vi "DriveModuleControl_TravTuneKsKv.vi"(8 "error in":errorcluster, 9 "Actual State":T1={"Speed"=0.0, "Angle"={"VALUE"=0.0, "COS"=1.0, "SIN"=0.0}} {"Angle"."SIN" format="%13.4f"; "Angle"."COS" format="%13.4f"; "Angle"."VALUE" format="%13.4f"}, 10 "Desired State":T1={"Speed"=0.0, "Angle"={"VALUE"=0.0, "COS"=1.0, "SIN"=0.0}} {"Angle"."SIN" format="%13.4f"; "Angle"."COS" format="%13.4f"; "Angle"."VALUE" format="%13.4f"}, 11 "ModualNamePrefix":i32) -> (0 "error out":errorcluster)   [LabVIEW 2020]
uses:
  <vilib>/Rock Robotics/WPI/ThirdParty/JAS_Junk/TrajLib/TypeDef/SWERVE_DRIVE_MODULE_STATE.ctl
  <vilib>/Rock Robotics/WPI/ThirdParty/JAS_Junk/TrajLib/TypeDef/ROTATION2D.ctl
  <vilib>/Rock Robotics/WPI/ThirdParty/JAS_Junk/TrajLib/Rotation2d_Minus.vi
  <vilib>/Rock Robotics/WPI/ThirdParty/JAS_Junk/TrajLib/Rotation2d_GetRadians.vi
  <vilib>/Rock Robotics/WPI/ThirdParty/JAS_Junk/TrajLib/SwerveModuleState_New.vi
  <vilib>/Rock Robotics/WPI/ThirdParty/JAS_Junk/TrajLib/Rotation2d_RotateBy.vi
  <vilib>/Rock Robotics/WPI/ThirdParty/JAS_Junk/TrajLib/Rotation2d_CreateAngle.vi
  <vilib>/Rock Robotics/WPI/ThirdParty/JAS_Junk/TrajLib/SimpleMotorFF_Calculate.vi
  <vilib>/Rock Robotics/WPI/ThirdParty/JAS_Junk/TrajLib/PIDController_AtSetpoint.vi
  <vilib>/Rock Robotics/WPI/ThirdParty/JAS_Junk/TrajLib/PIDController_SetPIDF.vi
  <vilib>/Rock Robotics/WPI/ThirdParty/JAS_Junk/TrajLib/PIDController_SetDerivativeFilter.vi
  <vilib>/Rock Robotics/WPI/ThirdParty/JAS_Junk/TrajLib/PIDController_SetIntegratorRange.vi
  <vilib>/Rock Robotics/WPI/ThirdParty/JAS_Junk/TrajLib/PIDController_SetTolerancePandV.vi
  <vilib>/Rock Robotics/WPI/ThirdParty/JAS_Junk/TrajLib/PIDController_DisableContinousInput.vi
  <vilib>/Rock Robotics/WPI/ThirdParty/JAS_Junk/TrajLib/PIDController_EnableContinousInput.vi
  <vilib>/Rock Robotics/WPI/ThirdParty/JAS_Junk/TrajLib/PIDController_Reset.vi
  <vilib>/Rock Robotics/WPI/ThirdParty/JAS_Junk/TrajLib/PIDController_New.vi
  <vilib>/Rock Robotics/WPI/ThirdParty/JAS_Junk/TrajLib/PIDController_SetOutputLimits.vi
  <vilib>/Rock Robotics/WPI/ThirdParty/JAS_Junk/TrajLib/LinearFilter_ResetToValue.vi
  <vilib>/Rock Robotics/WPI/ThirdParty/JAS_Junk/TrajLib/LinearFilter_Calculate.vi
  <vilib>/Rock Robotics/WPI/ThirdParty/JAS_Junk/TrajLib/Rotation2d_UnaryMinus.vi
  <vilib>/Rock Robotics/WPI/ThirdParty/JAS_Junk/TrajLib/Rotation2d_CreateXY.vi
  <vilib>/Rock Robotics/WPI/ThirdParty/JAS_Junk/TrajLib/PIDController_NewPeriod.vi
  <vilib>/Rock Robotics/WPI/ThirdParty/JAS_Junk/TrajLib/Util_CalcDist.vi
  <vilib>/Rock Robotics/SystemInterfaces/NetworkCommunication/NetComm_UsageReport_report.vi
  DriveGlobal.vi
  <vilib>/Rock Robotics/WPI/ThirdParty/JAS_Junk/TrajLib/LinearFilter_MovingAverage.vi
  <vilib>/Rock Robotics/WPI/ThirdParty/JAS_Junk/TrajLib/LinearFilter_LowPassBW1.vi
  <vilib>/Rock Robotics/WPI/ThirdParty/JAS_Junk/TrajLib/LinearFilter_LowPassBW2.vi
  <vilib>/Rock Robotics/WPI/ThirdParty/JAS_Junk/TrajLib/LinearFilter_HighPassBW1.vi
  <vilib>/Rock Robotics/WPI/ThirdParty/JAS_Junk/TrajLib/LinearFilter_HighPassBW2.vi
  <vilib>/Rock Robotics/WPI/ThirdParty/JAS_Junk/TrajLib/Globals/Util_LibraryGlobals.vi
  <vilib>/Rock Robotics/WPI/ThirdParty/JAS_Junk/TrajLib/PIDController_AdvCalculate_FF_Sp_Pv.vi
  <vilib>/Utility/semaphor.llb/Obtain Semaphore Reference.vi
  <vilib>/Rock Robotics/WPI/ThirdParty/JAS_Junk/TrajLib/Timer_Reset.vi
  <vilib>/Rock Robotics/Network Tables/NT Write Number.vi
  <vilib>/Rock Robotics/WPI/ThirdParty/JAS_Junk/TrajLib/Trajectory_Library.lvlib
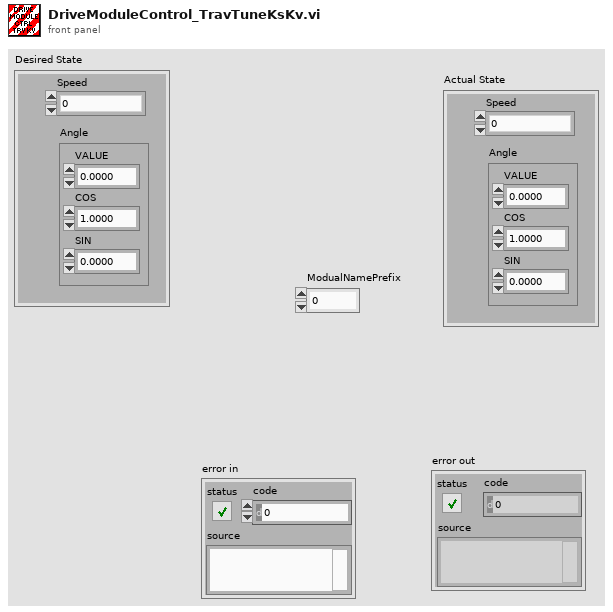
[diagram p1: front panel]
types:
  T1 = typedef "Trajectory_Library.lvlib/SWERVE_DRIVE_MODULE_STATE.ctl" = cluster{"Speed":dbl, "Angle":T2}
  T2 = typedef "Trajectory_Library.lvlib/ROTATION2D.ctl" = cluster{"VALUE":dbl, "COS":dbl, "SIN":dbl}
  T3 = enum16{"Moving Average", "Low Pass 1st Order Butterworth", "Low Pass 2nd Order Butterworth", "High Pass 1st Order Butterworth", "High Pass 2nd Order Butterworth"}
  T4 = typedef "WPI_MotorControlDeviceRef.ctl" = cluster{"DeviceStatus":errorcluster, "Type":T5, "PWM":cluster{"PWM Channel":T6, "DeadBand":T7}, "CAN":cluster{"Device Number":u8, "SetOutput VI Ref":variant, "GetOutput VI Ref":variant, "Enable VI Ref":variant, "Disable VI Ref":variant, "Data":variant}, "Invert":bool, "DIO PWM":cluster{"PWM \"Enable\" Channel":T6, "DIOChannel":T8, "PWM Rate":dbl}}
  T5 = typedef "WPI_MotorControlType.ctl" = enum16{"PWM", "CAN", "DIO PWM"}
  T6 = typedef "FPGA_DIOPWMChannel.ctl" = enum8{"PWM 0", "PWM 1", "PWM 2", "PWM 3", "PWM 4", "PWM 5", "PWM 6", "PWM 7", "PWM 8", "PWM 9", "PWM MXP 0", "PWM MXP 1", "PWM MXP 2", "PWM MXP 3", "PWM MXP 4", "PWM MXP 5", "PWM MXP 6", "PWM MXP 7", "PWM MXP 8", "PWM MXP 9", "Invalid"}
  T7 = typedef "WPI_PWMDeadband.ctl" = cluster{"Name":string, "maxPositivePwm":i32, "minPositivePwm":i32, "centerPwm":i32, "maxNegativePwm":i32, "minNegativePwm":i32, "angularRange":u16}
  T8 = typedef "FPGA_DIOChannel.ctl" = enum8{"DIO 0", "DIO 1", "DIO 2", "DIO 3", "DIO 4", "DIO 5", "DIO 6", "DIO 7", "DIO 8", "DIO 9", "DIO MXP 0", "DIO MXP 1", "DIO MXP 2", "DIO MXP 3", "DIO MXP 4", "DIO MXP 5", "DIO MXP 6", "DIO MXP 7", "DIO MXP 8", "DIO MXP 9", "DIO MXP 10", "DIO MXP 11", "DIO MXP 12", "DIO MXP 13", "DIO MXP 14", "DIO MXP 15", "SPI Port CS1", "SPI Port CS2", "SPI Port CS3", "SPI Port MISO", "SPI Port MOSI", "Invalid"}
  T9 = typedef "Trajectory_Library.lvlib/TIMER.ctl" = cluster{"StartTime":dbl, "Accumulated TIme":dbl, "Running":bool, "semaphore":T10}
  T10 = typedef "Semaphore RefNum" = refnum<k1>
  T11 = typedef "Trajectory_Library.lvlib/SIMPLE_MOTOR_FF.ctl" = cluster{"Ks":dbl, "Kv":dbl, "Ka":dbl, "KnInv":dbl}
  T12 = typedef "Trajectory_Library.lvlib/PID_ADV_LIMITS.ctl" = cluster{"MaxInput":dbl, "MinInput":dbl, "Continuous":bool, "MaxOutput":dbl, "MinOutput":dbl}
  T13 = typedef "Trajectory_Library.lvlib/PID_ADV_TUNING.ctl" = cluster{"Kf":dbl, "Kp":dbl, "Ki":dbl, "Kd":dbl, "MaximumIntegral":dbl, "MinimumIntegral":dbl, "Filter Derivative":bool}
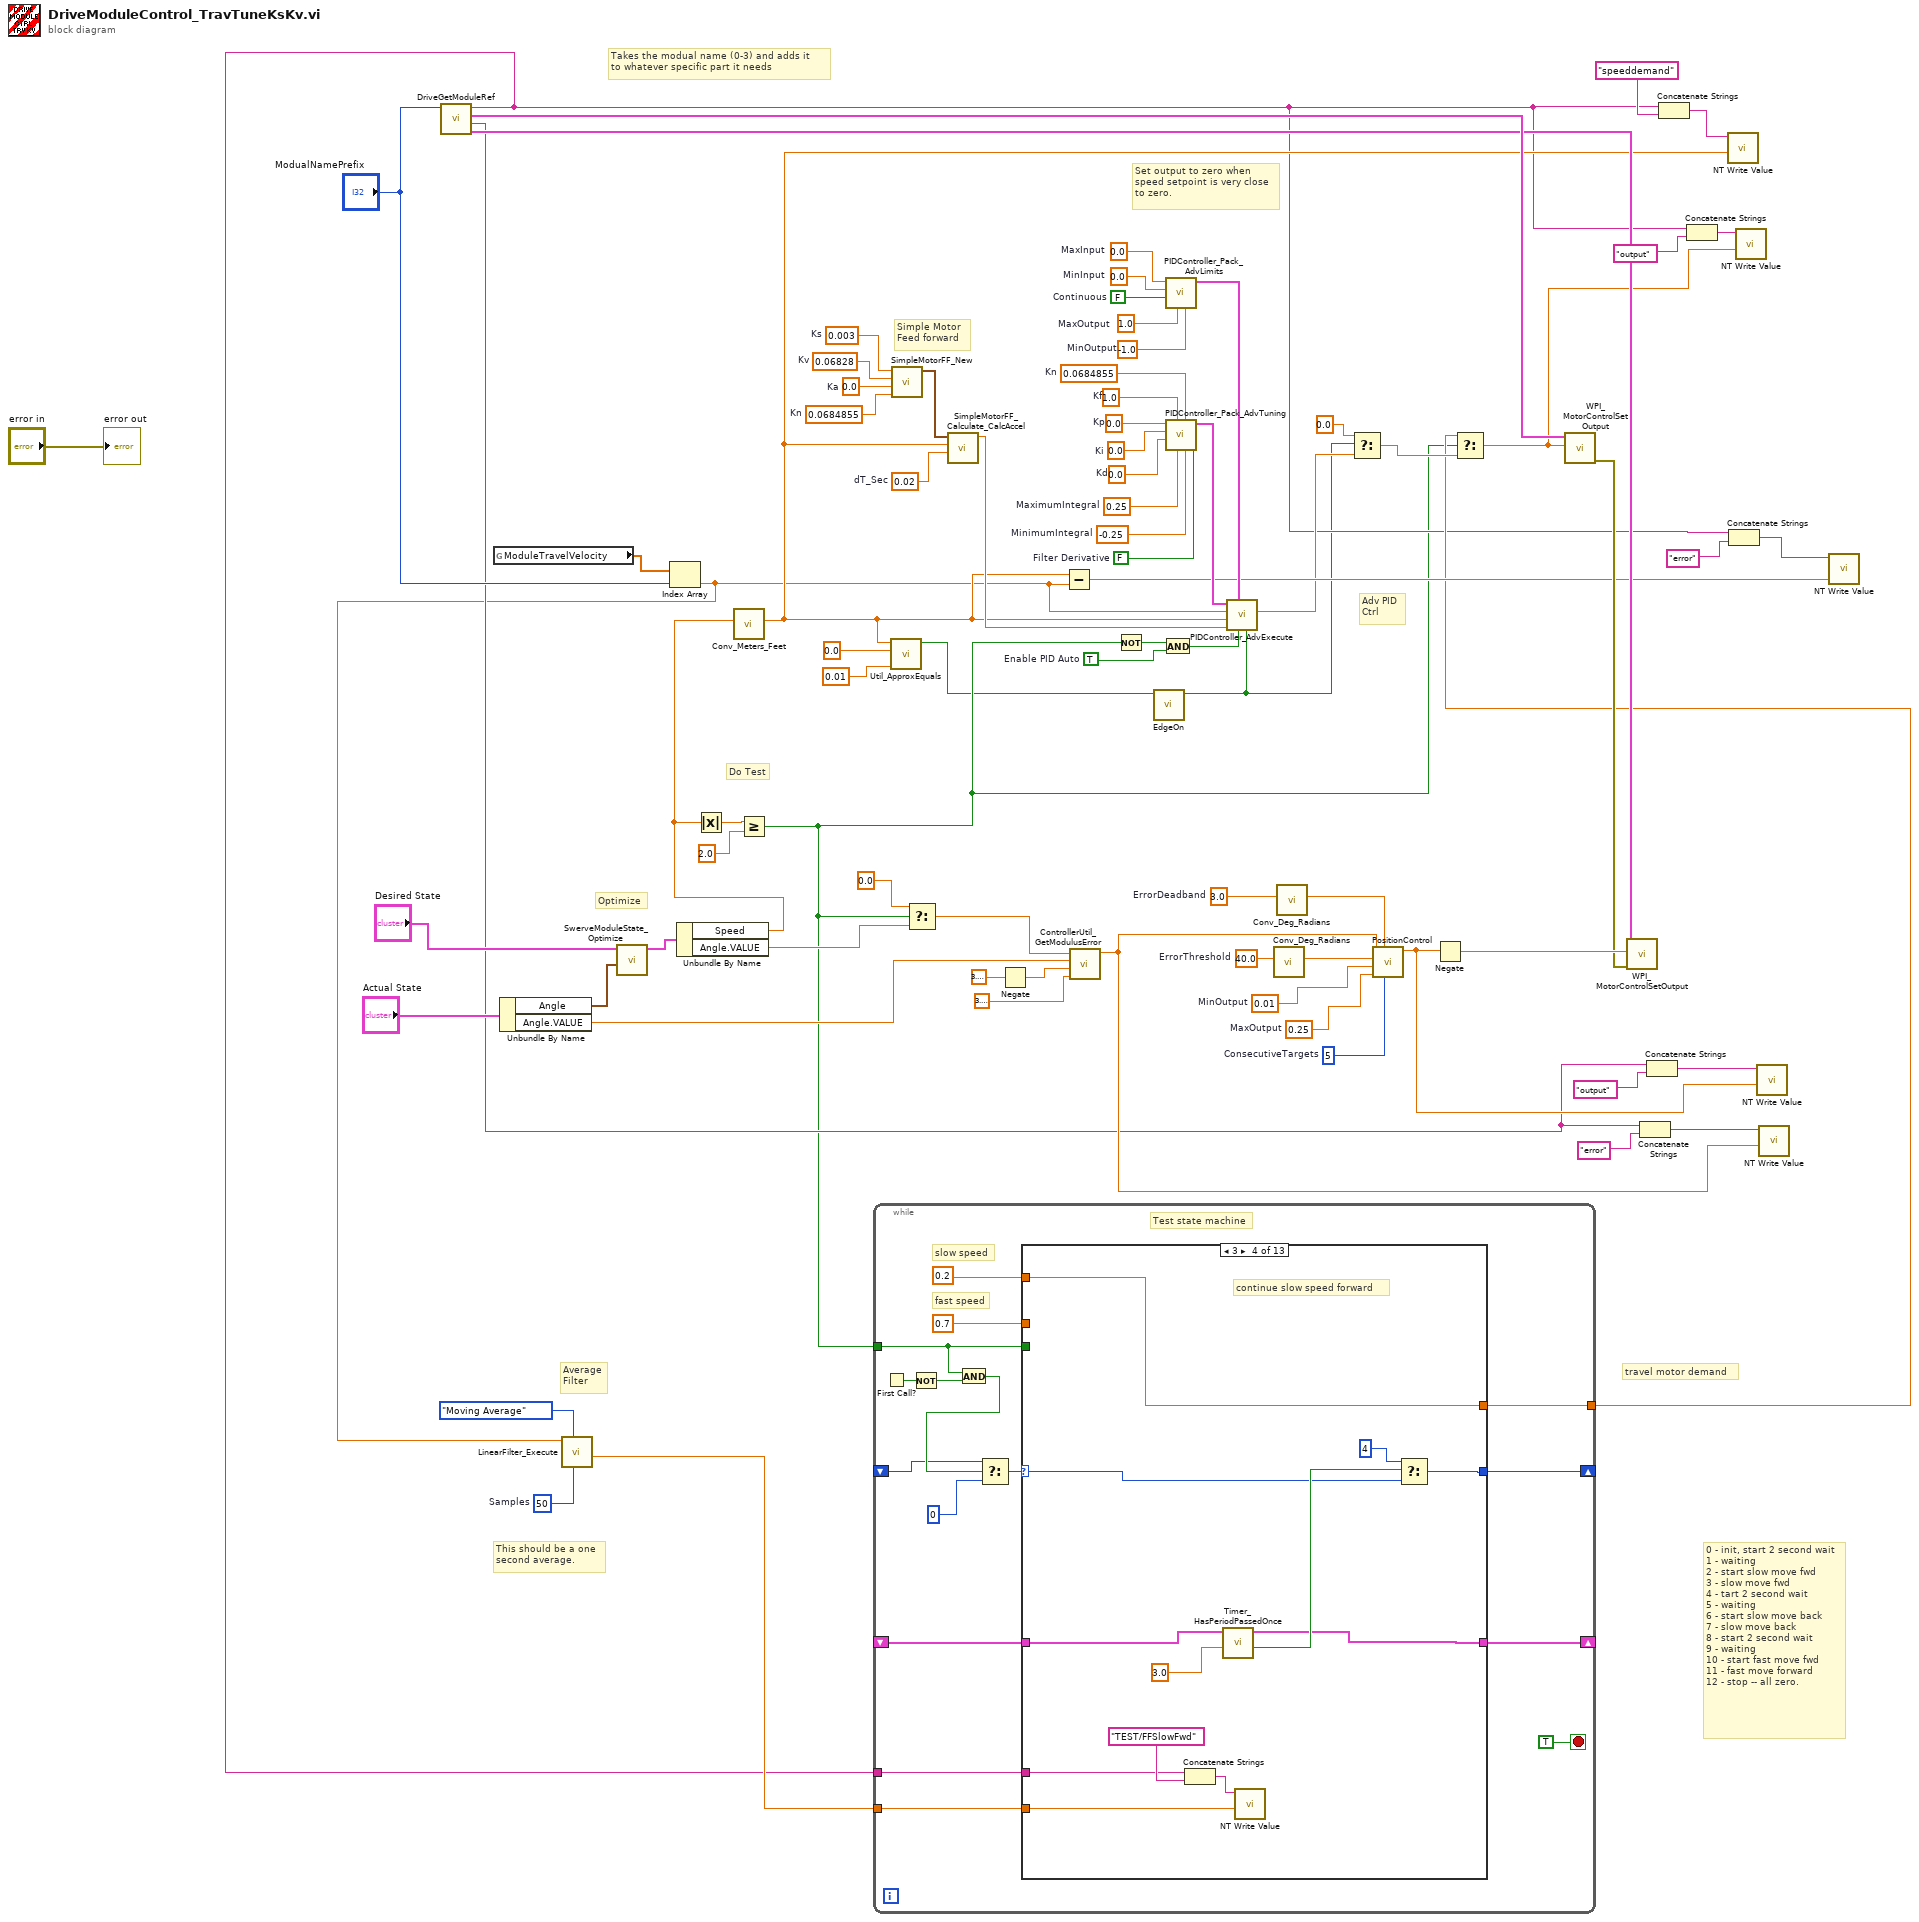
[diagram p0: block diagram]
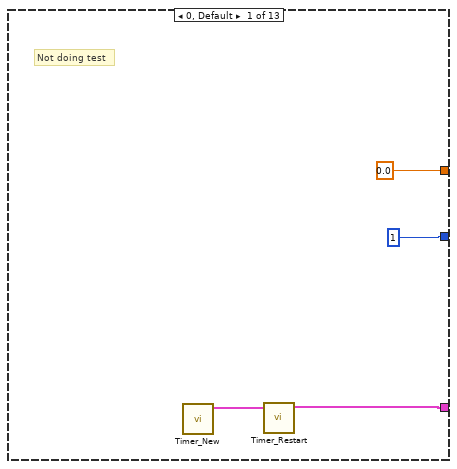
[diagram p2: hidden frame]
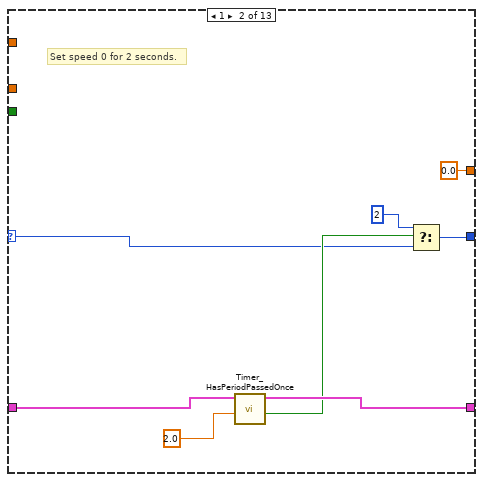
[diagram p3: hidden frame]
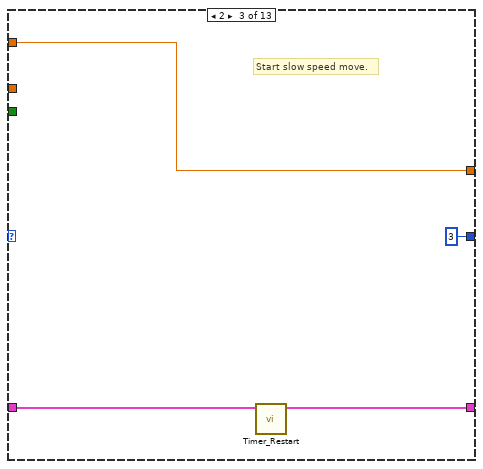
[diagram p4: hidden frame]
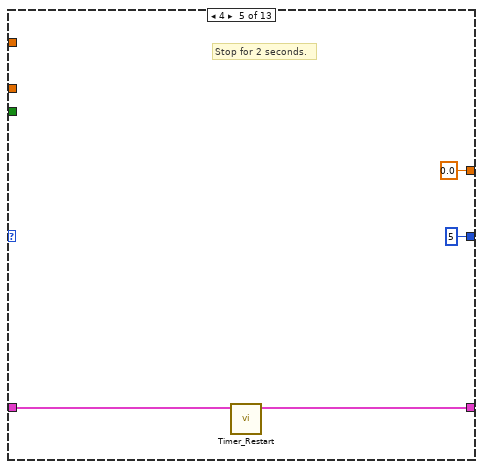
[diagram p5: hidden frame]
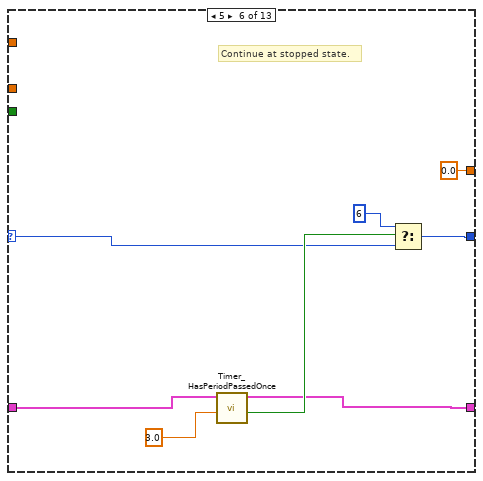
[diagram p6: hidden frame]
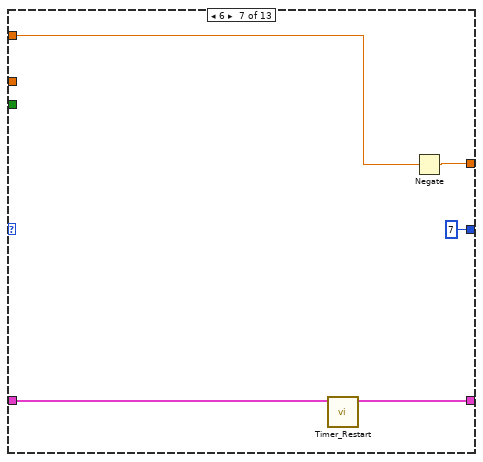
[diagram p7: hidden frame]
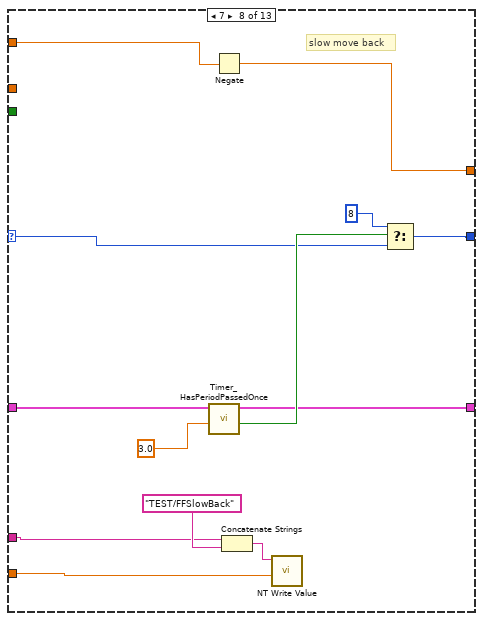
[diagram p8: hidden frame]
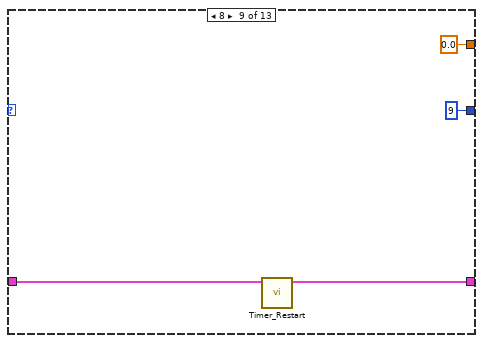
[diagram p9: hidden frame]
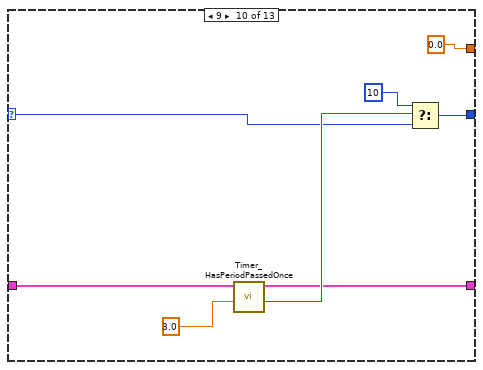
[diagram p10: hidden frame]
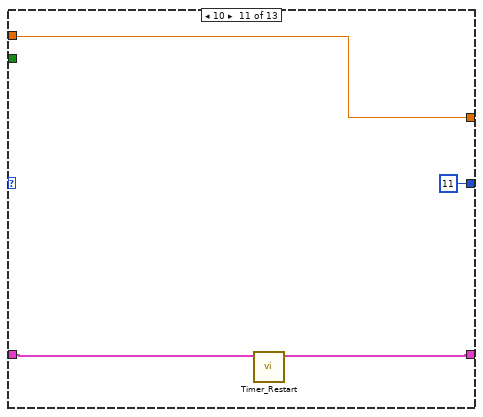
[diagram p11: hidden frame]
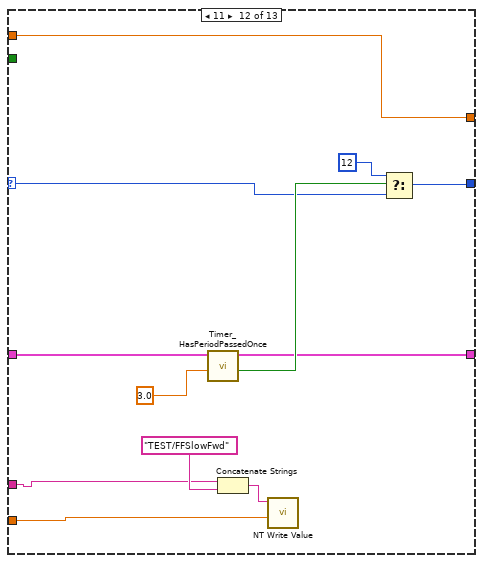
[diagram p12: hidden frame]
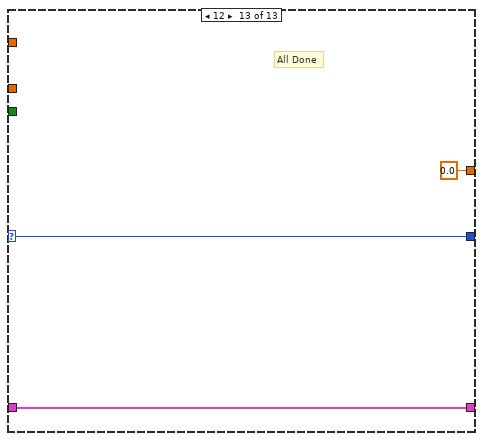
[diagram p13: hidden frame]
diagram:
  w8 = 50  # Samples
  w20 = TRUE  # Enable PID Auto
  w30 = 0.0684855  # Kn
  w47 = 0.0  # Kp
  w46 = 0.0  # Ki
  w45 = 0.0  # Kd
  w44 = 1.0  # Kf
  w43 = 0.25  # MaximumIntegral
  w42 = -0.25  # MinimumIntegral
  w41 = FALSE  # Filter Derivative
  w39 = 0.0  # MinInput
  w38 = FALSE  # Continuous
  w37 = 1.0  # MaxOutput
  w40 = -1.0  # MinOutput
  w36 = 0.0  # MaxInput
  w56 = 0.0684855  # Kn
  w55 = 0.02  # dT_Sec
  w53 = 0.003  # Ks
  w52 = 0.06828  # Kv
  w51 = 0.0  # Ka
  w66 = 5  # ConsecutiveTargets
  w63 = 0.25  # MaxOutput
  w67 = 0.01  # MinOutput
  w60 = 40.0  # ErrorThreshold
  w62 = 3.0  # ErrorDeadband
  # "This should be a one\nsecond average."
  # "Average\nFilter"
  # "0 - init, start 2 second wait\n1 - waiting\n2 - start slow move fwd\n3 - slow move fwd\n4 - tart 2 second wait\n5 - waiting\n6 - start slow move back\n7 - slow move back\n8 - start 2 second wait\n9 - waiting\n10 - start fast move fwd\n11 - fast move forward\n12 - stop -- all zero."
  # "travel motor demand"
  # "Do Test"
  # "Optimize"
  # "Set output to zero when\nspeed setpoint is very close\nto zero."
  # "Adv PID\nCtrl"
  # "Simple Motor\nFeed forward"
  # "Takes the modual name (0-3) and adds it \nto whatever specific part it needs"
  n1 = call "DriveGetModuleRef.vi"("ModualNamePrefix"="ModualNamePrefix") -> ("SpinMot"=w48:T4, "SpinStr"=w26:string, "TravMot"=w49:T4, "TravStr"=w4:string)  [unwired: 5 in, 2 out]
  n2 = global read "DriveGlobal.vi" "ModuleTravelVelocity"() -> (w32:dbl[])
  n3 = Unbundle By Name("Actual State") -> ("Angle"=w73:T2, "Angle.VALUE"=w70:dbl)
  n4 = call <vilib>:"SwerveModuleState_Optimize.vi"("CurrentAngle"=w73, "Desired State"="Desired State") -> ("out SWERVE_DRIVE_MODULE_STATE"=w71:T1)  [unwired: 9 in]
  n5 = Index Array(array=w32, index="ModualNamePrefix") -> (element=w6:dbl)
  n6 = call <vilib>:"LinearFilter_Execute.vi"("Samples"=w8, "Filter Type"=T3."Moving Average", "Input"=w6) -> ("Output"=w5:dbl)  [unwired: 7 in, 1 out]
  n7 = Unbundle By Name(w71) -> ("Speed"=w17:dbl, "Angle.VALUE"=w14:dbl)
  n8 = Absolute Value(x=w17) -> (abs(x)=w16:dbl)
  n9 = call <vilib>:"Conv_Meters_Feet.vi"("Meters"=w17) -> ("Feet"=w23:dbl)  [unwired: 10 in]
  n10 = Greater Or Equal?(x=w16, y=2.0) -> (x >= y?=w3:bool)
  n11 = while {
    shift-right: [w98] -> _
    shift-left: _ -> [w90]
    shift-right: [w97] -> _
    shift-left: _ -> [w88]
    tunnel: w3 -> [w92]
    tunnel: [w89] -> w9
    tunnel: w5 -> [w85]
    tunnel: w4 -> [w84]
    stop <- TRUE stop-if-true
    # "fast speed"
    # "slow speed"
    # "Test state machine"
    n12 = First Call?() -> (First Call?: T/F=w94:bool)
    n13 = Not(x=w94) -> (.not. x?=w93:bool)
    n14 = And(x=w92, y=w93) -> (x .and. y?=w91:bool)
    n15 = Select(t=w90, s=w91, f=0 ("t")) -> (s? t:f=w96:i32)
    n16 = case shown="3" w96 {
      selector: w96 -> [_ w106 _ w123 _ w135 _ w151 _ w162 _ w178 w187]
      tunnel: [1 w105 3 ("t") w124 5 ("t") w136 7 ("t") w152 9 ("t") w166 11 ("t") w181 w187] -> w98
      tunnel: [w102 w109 w113 w121 w129 w133 w144 w149 w159 w164 w170 w179 w186] -> w97
      tunnel: w92 -> [_ _ _ _ _ _ _ _ _ _ _ _ _]
      tunnel: [0.0 0.0 w112 w120 0.0 0.0 w141 w156 0.0 0.0 w173 w185 0.0] -> w89
      tunnel: w88 -> [_ w110 w114 w122 w130 w134 w143 w150 w158 w165 w171 w180 w186]
      tunnel: 0.2 -> [_ _ w112 w120 _ _ w140 w157 _ _ _ _ _]
      tunnel: 0.7 -> [_ _ _ _ _ _ _ _ _ _ w173 w185 _]
      tunnel: w85 -> [_ _ _ w119 _ _ _ w145 _ _ _ w174 _]
      tunnel: w84 -> [_ _ _ w116 _ _ _ w146 _ _ _ w175 _]
      frame 0, Default {
        # "Not doing test"
        n17 = call <vilib>:"Timer_New.vi"() -> ("TIMER"=w103:T9)  [unwired: 11 in]
        n18 = call <vilib>:"Timer_Restart.vi"("in Timer"=w103) -> ("out Timer"=w102:T9)  [unwired: 10 in]
      }
      frame 1 {
        # "Set speed 0 for 2 seconds."
        n19 = call <vilib>:"Timer_HasPeriodPassedOnce.vi"("Period"=2.0, "in Timer"=w110) -> ("Expired"=w107:bool, "out Timer"=w109:T9)  [unwired: 7 in, 1 out]
        n20 = Select(t=2, s=w107, f=w106) -> (s? t:f=w105:i32)
      }
      frame 2 {
        # "Start slow speed move."
        n21 = call <vilib>:"Timer_Restart.vi"("in Timer"=w114) -> ("out Timer"=w113:T9)  [unwired: 10 in]
      }
      frame 3 {
        # "continue slow speed forward"
        n22 = Concatenate Strings(w116, "TEST/FFSlowFwd" ("refnum name")) -> (w117:string)
        n23 = call <vilib>:"Timer_HasPeriodPassedOnce.vi"("Period"=3.0, "in Timer"=w122) -> ("Expired"=w126:bool, "out Timer"=w121:T9)  [unwired: 7 in, 1 out]
        n24 = call-poly <vilib>:"NT Write Value.vi"("value"=w119, "name"=w117) -> ()  [unwired: 9 in, 1 out]
        n25 = Select(t=4, s=w126, f=w123) -> (s? t:f=w124:i32)
      }
      frame 4 {
        # "Stop for 2 seconds."
        n26 = call <vilib>:"Timer_Restart.vi"("in Timer"=w130) -> ("out Timer"=w129:T9)  [unwired: 10 in]
      }
      frame 5 {
        # "Continue at stopped state."
        n27 = call <vilib>:"Timer_HasPeriodPassedOnce.vi"("Period"=3.0, "in Timer"=w134) -> ("Expired"=w138:bool, "out Timer"=w133:T9)  [unwired: 7 in, 1 out]
        n28 = Select(t=6, s=w138, f=w135) -> (s? t:f=w136:i32)
      }
      frame 6 {
        n29 = call <vilib>:"Timer_Restart.vi"("in Timer"=w143) -> ("out Timer"=w144:T9)  [unwired: 10 in]
        n30 = Negate(x=w140) -> (-x=w141:dbl)
      }
      frame 7 {
        # "slow move back"
        n31 = call <vilib>:"Timer_HasPeriodPassedOnce.vi"("Period"=3.0, "in Timer"=w150) -> ("Expired"=w154:bool, "out Timer"=w149:T9)  [unwired: 7 in, 1 out]
        n32 = Negate(x=w157) -> (-x=w156:dbl)
        n33 = Concatenate Strings(w146, "TEST/FFSlowBack" ("refnum name")) -> (w147:string)
        n34 = call-poly <vilib>:"NT Write Value.vi"("value"=w145, "name"=w147) -> ()  [unwired: 9 in, 1 out]
        n35 = Select(t=8, s=w154, f=w151) -> (s? t:f=w152:i32)
      }
      frame 8 {
        n36 = call <vilib>:"Timer_Restart.vi"("in Timer"=w158) -> ("out Timer"=w159:T9)  [unwired: 10 in]
      }
      frame 9 {
        n37 = call <vilib>:"Timer_HasPeriodPassedOnce.vi"("Period"=3.0, "in Timer"=w165) -> ("Expired"=w168:bool, "out Timer"=w164:T9)  [unwired: 7 in, 1 out]
        n38 = Select(t=10, s=w168, f=w162) -> (s? t:f=w166:i32)
      }
      frame 10 {
        n39 = call <vilib>:"Timer_Restart.vi"("in Timer"=w171) -> ("out Timer"=w170:T9)  [unwired: 10 in]
      }
      frame 11 {
        n40 = call <vilib>:"Timer_HasPeriodPassedOnce.vi"("Period"=3.0, "in Timer"=w180) -> ("Expired"=w183:bool, "out Timer"=w179:T9)  [unwired: 7 in, 1 out]
        n41 = Concatenate Strings(w175, "TEST/FFSlowFwd" ("refnum name")) -> (w176:string)
        n42 = call-poly <vilib>:"NT Write Value.vi"("value"=w174, "name"=w176) -> ()  [unwired: 9 in, 1 out]
        n43 = Select(t=12, s=w183, f=w178) -> (s? t:f=w181:i32)
      }
      frame 12 {
        # "All Done"
      }
    }
  }
  n44 = call <vilib>:"Util_ApproxEquals.vi"("Tolerance"=0.01, "Value 2"=0.0, "Value 1"=w23) -> ("ApproxEquals"=w2:bool)  [unwired: 8 in]
  n45 = call <vilib>:"SimpleMotorFF_New.vi"("Kn"=w56, "Ka"=w51, "Kv"=w52, "Ks"=w53) -> ("SIMPLE_MOTOR_FF"=w54:T11)  [unwired: 7 in]
  n46 = Select(t=0.0, s=w3, f=w14) -> (s? t:f=w10:dbl)
  n47 = call <vilib>:"SimpleMotorFF_Calculate_CalcAccel.vi"("dT_Sec"=w55, "VelSp"=w23, "SIMPLE_MOTOR_FF"=w54) -> ("FeedForward"=w33:dbl)  [unwired: 8 in]
  n48 = Negate(x=3.141592653589793) -> (-x=w72:dbl)
  n49 = Subtract(x=w23, y=w6) -> (x-y=w27:dbl)
  n50 = call <vilib>:"ControllerUtil_GetModulusError.vi"("Maximum_Input"=3.141592653589793, "Minimum_Input"=w72, "Measurerment(PV)"=w70, "Reference(SP)"=w10) -> ("Error"=w64:dbl)  [unwired: 7 in]
  n51 = Not(x=w3) -> (.not. x?=w21:bool)
  n52 = call "EdgeOn.vi"("Current State"=w2) -> ("Edge On Found"=w1:bool)  [unwired: 10 in]
  n53 = And(x=w21, y=w20) -> (x .and. y?=w22:bool)
  n54 = call <vilib>:"PIDController_Pack_AdvLimits.vi"("MinOutput"=w40, "MaxOutput"=w37, "Continuous"=w38, "MinInput"=w39, "MaxInput"=w36) -> ("Adv PID Limits"=w34:T12)  [unwired: 6 in]
  n55 = call <vilib>:"PIDController_Pack_AdvTuning.vi"("Filter Derivative"=w41, "MinimumIntegral"=w42, "Kn"=w30, "MaximumIntegral"=w43, "Kf"=w44, "Kd"=w45, "Ki"=w46, "Kp"=w47) -> ("Adv PID Tuning"=w35:T13)  [unwired: 3 in]
  n56 = call <vilib>:"PIDController_AdvExecute.vi"("Reset"=w1, "Auto"=w22, "Adv PID Limits"=w34, "FF-FeedForward"=w33, "SP-SetPoint"=w23, "PV-Measurement"=w6, "Adv PID Tuning"=w35) -> ("CO-ControlOutput"=w19:dbl)  [unwired: 2 in, 2 out]
  n57 = call <vilib>:"Conv_Deg_Radians.vi"("Degress"=w60) -> ("Radians"=w59:dbl)  [unwired: 10 in]
  n58 = call <vilib>:"Conv_Deg_Radians.vi"("Degress"=w62) -> ("Radians"=w61:dbl)  [unwired: 10 in]
  n59 = Select(t=0.0, s=w1, f=w19) -> (s? t:f=w11:dbl)
  n60 = call "PositionControl.vi"("ConsecutiveTargets"=w66, "ErrorDeadband"=w61, "MaxOutput"=w63, "MinOutput"=w67, "ErrorThreshold"=w59, "Error"=w64) -> ("OutputValue"=w58:dbl)  [unwired: 3 in, 2 out]
  n61 = Negate(x=w58) -> (-x=w57:dbl)
  n62 = Select(t=w9, s=w3, f=w11) -> (s? t:f=w12:dbl)
  n63 = call <vilib>:"WPI_MotorControlSetOutput.vi"("Output"=w12, "MotorControlDevRef"=w49) -> ("error out"=w50:errorcluster)  [unwired: 7 in, 2 out]
  n64 = call <vilib>:"WPI_MotorControlSetOutput.vi"("error in (no error)"=w50, "Output"=w57, "MotorControlDevRef"=w48) -> ()  [unwired: 6 in, 3 out]
  n65 = Concatenate Strings(w26, "error" ("refnum name")) -> (w77:string)
  n66 = Concatenate Strings(w26, "output" ("refnum name")) -> (w65:string)
  n67 = Concatenate Strings(w4, "speeddemand" ("refnum name")) -> (w81:string)
  n68 = Concatenate Strings(w4, "output" ("refnum name")) -> (w79:string)
  n69 = call-poly <vilib>:"NT Write Value.vi"("value"=w23, "name"=w81) -> ()  [unwired: 9 in, 1 out]
  n70 = Concatenate Strings(w4, "error" ("refnum name")) -> (w28:string)
  n71 = call-poly <vilib>:"NT Write Value.vi"("value"=w12, "name"=w79) -> ()  [unwired: 9 in, 1 out]
  n72 = call-poly <vilib>:"NT Write Value.vi"("value"=w58, "name"=w65) -> ()  [unwired: 9 in, 1 out]
  n73 = call-poly <vilib>:"NT Write Value.vi"("value"=w64, "name"=w77) -> ()  [unwired: 9 in, 1 out]
  n74 = call-poly <vilib>:"NT Write Value.vi"("value"=w27, "name"=w28) -> ()  [unwired: 9 in, 1 out]
  "error out" <- "error in"
